vi "flywheel.vi"(2 "Flywheel Button":bool, 3 "Flywheel PIDF":T1, 4 "kV":dbl, 8 "kS":dbl, 9 "Flywheel Setpoint RPM":dbl=4000.0) -> (7 "output graph":cluster{"RPM":dbl, "Flywheel Setpoint RPM":dbl})   [LabVIEW 2020]
uses:
  <vilib>/Rock Robotics/WPI/ThirdParty/Phoenix-LabVIEW/Motor Controller/Controls/CTRE_Phoenix_MotorControl_ControlMode.ctl
  <vilib>/Rock Robotics/WPI/ThirdParty/Phoenix-LabVIEW/Motor Controller/Get/CTRE_Phoenix_MotorController_GetSupplyAndStatorCurrent_Enhanced.vi
  <vilib>/Rock Robotics/WPI/ThirdParty/Phoenix-LabVIEW/Motor Controller/Get/CTRE_Phoenix_MotorController_GetSelectedSensorData.vi
  TitanLib/Lib/RawUnitsToRPM-2048-CPR.vi
  TitanLib/Lib/TitanLib.lvlib
  TitanLib/Lib/RPMToRawUnits-2048-CPR.vi
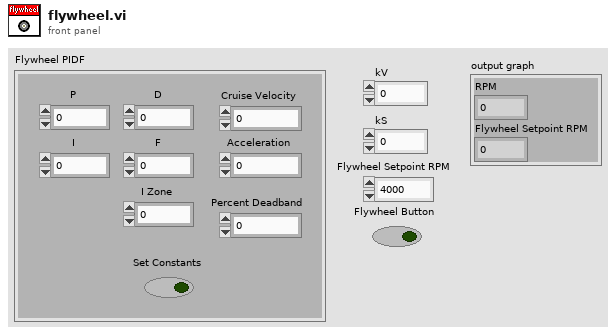
[diagram p1: front panel]
types:
  T1 = cluster{"Set Constants":bool, "P":dbl, "I":dbl, "D":dbl, "F":dbl, "I Zone":dbl, "Cruise Velocity":i32, "Acceleration":i32, "Percent Deadband":dbl}
  T2 = typedef "WPI_MotorControlDeviceRef.ctl" = cluster{"DeviceStatus":errorcluster, "Type":T3, "PWM":cluster{"PWM Channel":T4, "DeadBand":T5}, "CAN":cluster{"Device Number":u8, "SetOutput VI Ref":variant, "GetOutput VI Ref":variant, "Enable VI Ref":variant, "Disable VI Ref":variant, "Data":variant}, "Invert":bool, "DIO PWM":cluster{"PWM \"Enable\" Channel":T4, "DIOChannel":T6, "PWM Rate":dbl}}
  T3 = typedef "WPI_MotorControlType.ctl" = enum16{"PWM", "CAN", "DIO PWM"}
  T4 = typedef "FPGA_DIOPWMChannel.ctl" = enum8{"PWM 0", "PWM 1", "PWM 2", "PWM 3", "PWM 4", "PWM 5", "PWM 6", "PWM 7", "PWM 8", "PWM 9", "PWM MXP 0", "PWM MXP 1", "PWM MXP 2", "PWM MXP 3", "PWM MXP 4", "PWM MXP 5", "PWM MXP 6", "PWM MXP 7", "PWM MXP 8", "PWM MXP 9", "Invalid"}
  T5 = typedef "WPI_PWMDeadband.ctl" = cluster{"Name":string, "maxPositivePwm":i32, "minPositivePwm":i32, "centerPwm":i32, "maxNegativePwm":i32, "minNegativePwm":i32, "angularRange":u16}
  T6 = typedef "FPGA_DIOChannel.ctl" = enum8{"DIO 0", "DIO 1", "DIO 2", "DIO 3", "DIO 4", "DIO 5", "DIO 6", "DIO 7", "DIO 8", "DIO 9", "DIO MXP 0", "DIO MXP 1", "DIO MXP 2", "DIO MXP 3", "DIO MXP 4", "DIO MXP 5", "DIO MXP 6", "DIO MXP 7", "DIO MXP 8", "DIO MXP 9", "DIO MXP 10", "DIO MXP 11", "DIO MXP 12", "DIO MXP 13", "DIO MXP 14", "DIO MXP 15", "SPI Port CS1", "SPI Port CS2", "SPI Port CS3", "SPI Port MISO", "SPI Port MOSI", "Invalid"}
  T7 = typedef "CTRE_Phoenix_MotorControl_ControlMode.ctl" = u16
  T8 = enum16{"DemandType_Neutral", "DemandType_AuxPID", "DemandType_ArbitraryFeedForward"}
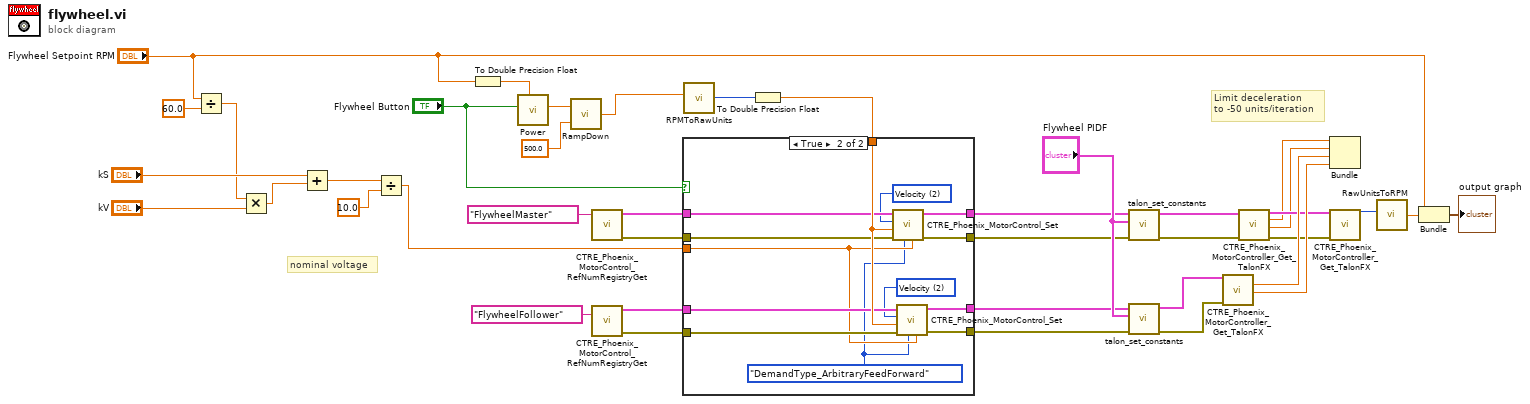
[diagram p0: block diagram]
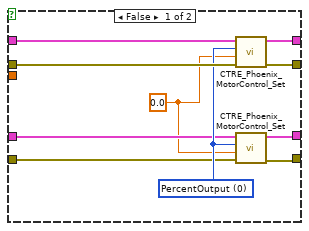
[diagram p2: hidden frame]
diagram:
  # "Limit deceleration\nto -50 units/iteration"
  # "nominal voltage"
  n1 = Divide(x="Flywheel Setpoint RPM", y=60.0) -> (x/y=w14:dbl)
  n2 = Multiply(x=w14, y="kV") -> (x*y=w28:dbl)
  n3 = Add(x="kS", y=w28) -> (x+y=w29:dbl)
  n4 = Divide(x=w29, y=10.0) -> (x/y=w31:dbl)
  n5 = To Double Precision Float(number="Flywheel Setpoint RPM") -> (double precision float=w17:dbl)
  n6 = call "Power.vi"("Positive Power"=w17, "Positive"="Flywheel Button") -> ("Output"=w24:dbl)  [unwired: 9 in]
  n7 = call "RampDown.vi"("Decrease per Cycle"=500.0, "Input"=w24) -> ("Output"=w3:dbl)
  n8 = call <vilib>:"CTRE_Phoenix_MotorControl_RefNumRegistryGet.vi"("refnum name"="FlywheelMaster") -> ("error out"=w21:errorcluster, "PhoenixMotorControlDevRef"=w20:T2)  [unwired: 9 in]
  n9 = call <vilib>:"CTRE_Phoenix_MotorControl_RefNumRegistryGet.vi"("refnum name"="FlywheelFollower") -> ("error out"=w23:errorcluster, "PhoenixMotorControlDevRef"=w22:T2)  [unwired: 9 in]
  n10 = call-poly "RPMToRawUnits.vi"("RPM"=w3) -> ("Raw Units"=w2:i32)  [unwired: 3 in]
  n11 = To Double Precision Float(number=w2) -> (double precision float=w1:dbl)
  n12 = case shown="True" "Flywheel Button" {
    tunnel: [w44 w63] -> w35
    tunnel: [w45 w62] -> w34
    tunnel: [w43 w61] -> w33
    tunnel: [w42 w60] -> w32
    tunnel: w31 -> [_ w52]
    tunnel: w1 -> [_ w59]
    tunnel: w23 -> [w46 w58]
    tunnel: w22 -> [w47 w57]
    tunnel: w21 -> [w50 w55]
    tunnel: w20 -> [w49 w54]
    frame False {
      w41 = 0.0 ("Output")
      w48 = T7 0 items=["PercentOutput"=0, "Position"=1, "Velocity"=2, "Current"=3, "Follower"=5, "MotionProfile"=6, "MotionMagic"=7, "MotionProfileArc"=10, "Disabled"=15] ("Control Mode")
      n13 = call <vilib>:"CTRE_Phoenix_MotorControl_Set.vi"("error in (no error)"=w50, "Output"=w41, "Control Mode"=w48, "PhoenixMotorControlDevRef"=w49) -> ("error out"=w43:errorcluster, "PhoenixMotorControlDevRef"=w42:T2)  [unwired: 6 in]
      n14 = call <vilib>:"CTRE_Phoenix_MotorControl_Set.vi"("error in (no error)"=w46, "Output"=w41, "Control Mode"=w48, "PhoenixMotorControlDevRef"=w47) -> ("error out"=w44:errorcluster, "PhoenixMotorControlDevRef"=w45:T2)  [unwired: 6 in]
    }
    frame True {
      w51 = T8."DemandType_ArbitraryFeedForward" ("DemandType")
      w56 = T7 2 items=["PercentOutput"=0, "Position"=1, "Velocity"=2, "Current"=3, "Follower"=5, "MotionProfile"=6, "MotionMagic"=7, "MotionProfileArc"=10, "Disabled"=15] ("Control Mode")
      w53 = T7 2 items=["PercentOutput"=0, "Position"=1, "Velocity"=2, "Current"=3, "Follower"=5, "MotionProfile"=6, "MotionMagic"=7, "MotionProfileArc"=10, "Disabled"=15] ("Control Mode")
      n15 = call <vilib>:"CTRE_Phoenix_MotorControl_Set.vi"("Demand1"=w52, "DemandType"=w51, "error in (no error)"=w55, "Output"=w59, "Control Mode"=w53, "PhoenixMotorControlDevRef"=w54) -> ("error out"=w61:errorcluster, "PhoenixMotorControlDevRef"=w60:T2)  [unwired: 4 in]
      n16 = call <vilib>:"CTRE_Phoenix_MotorControl_Set.vi"("Demand1"=w52, "DemandType"=w51, "error in (no error)"=w58, "Output"=w59, "Control Mode"=w56, "PhoenixMotorControlDevRef"=w57) -> ("error out"=w63:errorcluster, "PhoenixMotorControlDevRef"=w62:T2)  [unwired: 4 in]
    }
  }
  n17 = call "talon_set_constants.vi"("error in"=w33, "Constants"="Flywheel PIDF", "PhoenixMotorControlDevRef"=w32) -> ("error out"=w38:errorcluster, "PhoenixMotorControlDevRef"=w37:T2)  [unwired: 7 in]
  n18 = call "talon_set_constants.vi"("error in"=w35, "Constants"="Flywheel PIDF", "PhoenixMotorControlDevRef"=w34) -> ("error out"=w40:errorcluster, "PhoenixMotorControlDevRef"=w39:T2)  [unwired: 7 in]
  n19 = call-poly <vilib>:"CTRE_Phoenix_MotorController_Get_TalonFX.vi"("PhoenixMotorControlDevRef"=w39, "error in"=w40) -> ("Supply Current"=w13:dbl, "Stator Current"=w12:dbl)  [unwired: 10 in, 2 out]
  n20 = call-poly <vilib>:"CTRE_Phoenix_MotorController_Get_TalonFX.vi"("PhoenixMotorControlDevRef"=w37, "error in"=w38) -> ("PhoenixMotorControlDevRef"=w11:T2, "Supply Current"=w9:dbl, "Stator Current"=w8:dbl, "error out"=w10:errorcluster)  [unwired: 10 in]
  n21 = Bundle("Supply Current"=w9, "Stator Current"=w8, "Supply Current"=w13, "Stator Current"=w12) -> ()  [unwired: 1 in, 1 out]
  n22 = call-poly <vilib>:"CTRE_Phoenix_MotorController_Get_TalonFX.vi"("PhoenixMotorControlDevRef"=w11, "error in"=w10) -> ("Velocity (Raw Sensor Units per 100 ms)"=w7:i32)  [unwired: 10 in, 3 out]
  n23 = call-poly "RawUnitsToRPM.vi"("Raw Units"=w7) -> ("RPM"=w6:dbl)  [unwired: 3 in]
  n24 = Bundle("RPM"=w6, "Flywheel Setpoint RPM"="Flywheel Setpoint RPM") -> (→"output graph":cluster{"RPM":dbl, "Flywheel Setpoint RPM":dbl})  [unwired: 1 in]
